vi "CIMAQ_Create_Grayscale.vi"   [LabVIEW 2017]
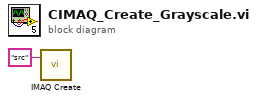
[diagram p0: block diagram]
diagram:
  n1 = call "IMAQ Create"("Image Name"="src") -> ()  [unwired: 4 in, 2 out]
